vi "ConfigurePerCellMotionAnalysis.vi"(4 "Scan Settings (um)":T1={"XStart"=1, "XEnd"=1, "XNum"=1, "YStart"=1, "YEnd"=1, "YNum"=1, "ZStart"=1, "ZEnd"=1, "ZNum"=1}, 5 "Points Selected":i32, 6 "Scan Settings":T1={"XStart"=1, "XEnd"=1, "XNum"=1, "YStart"=1, "YEnd"=1, "YNum"=1, "ZStart"=1, "ZEnd"=1, "ZNum"=1}, 7 "Sampling Structure":u16(ring) items=["Cube Vertices"], 8 "error in (no error)":errorcluster, 9 "Per Cell Motion Analysis":bool, 10 "In Points":i32[][](array[numeric]), 11 "AODAcq in":refnum<class "AODAcq.lvclass">) -> (0 "error out":errorcluster, 1 "Additional Points":i32, 2 "Out Points":i32[][](array[numeric]), 3 "AODAcq out":refnum<class "AODAcq.lvclass">)   [LabVIEW 2014, in "AODAcq.lvclass"]
uses:
  AODAcq.lvclass
  Cube Vertices.vi
panel:
  # "On"
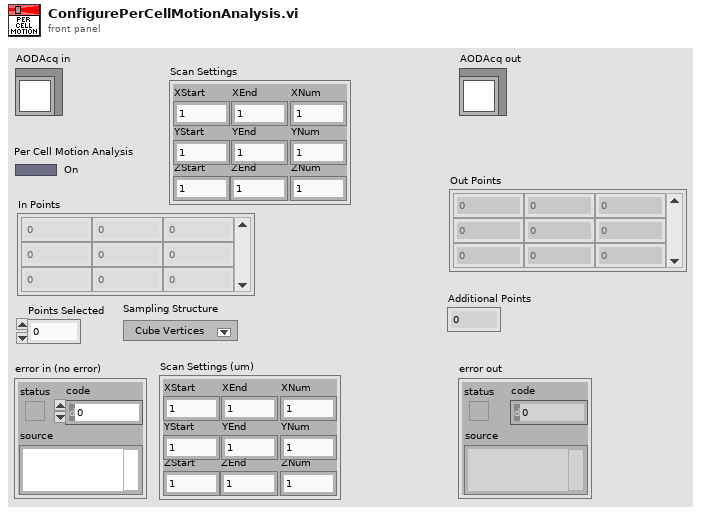
[diagram p1: front panel]
types:
  T1 = cluster{"XStart":i32, "XEnd":i32, "XNum":i32, "YStart":i32, "YEnd":i32, "YNum":i32, "ZStart":i32, "ZEnd":i32, "ZNum":i32}
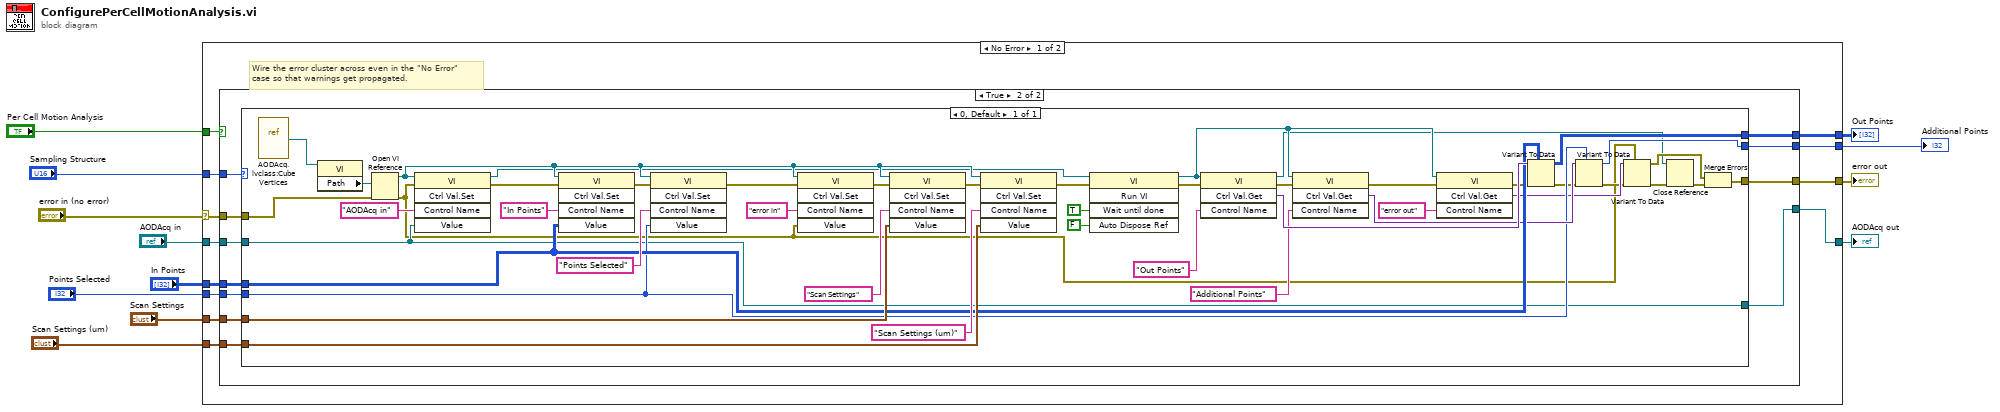
[diagram p0: block diagram]
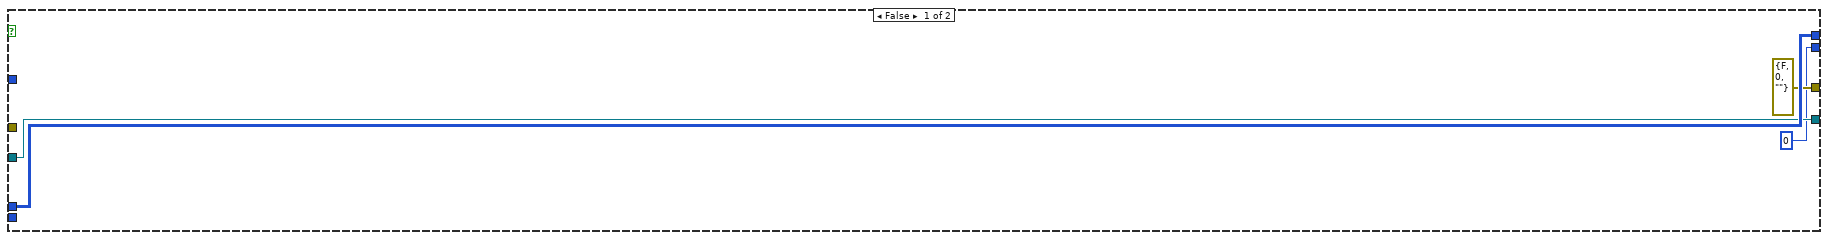
[diagram p2: hidden frame]
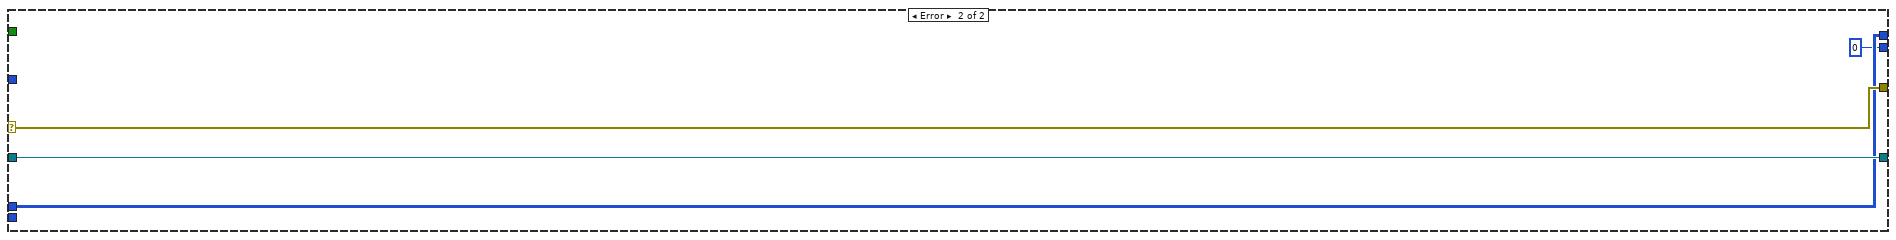
[diagram p3: hidden frame]
diagram:
  n1 = case shown="No Error" "error in (no error)" {
    selector: "error in (no error)" -> [w15 w88]
    tunnel: [w16 w88] -> w11
    tunnel: [w17 w87] -> w9
    tunnel: "AODAcq in" -> [w18 w87]
    tunnel: "Per Cell Motion Analysis" -> [w24 _]
    tunnel: "In Points" -> [w21 w86]
    tunnel: "Points Selected" -> [w23 _]
    tunnel: "Sampling Structure" -> [w22 _]
    tunnel: [w20 w86] -> w4
    tunnel: "Scan Settings" -> [w19 _]
    tunnel: "Scan Settings (um)" -> [w14 _]
    tunnel: [w13 0 ("Additional Points")] -> w1
    frame No Error {
      # "Wire the error cluster across even in the \"No Error\"\ncase so that warnings get propagated."
      n2 = case shown="True" w24 {
        tunnel: w23 -> [_ w39]
        tunnel: w22 -> [_ w38]
        tunnel: w21 -> [w28 w37]
        tunnel: [w28 w36] -> w20
        tunnel: w19 -> [_ w35]
        tunnel: w18 -> [w27 w34]
        tunnel: [w27 w29] -> w17
        tunnel: [errorcluster {"status"=FALSE, "code"=0, "source"=""} ("error out") w33] -> w16
        tunnel: w15 -> [_ w32]
        tunnel: w14 -> [_ w31]
        tunnel: [0 ("Additional Points") w30] -> w13
        frame False {
        }
        frame True {
          n3 = case shown="0, Default" w38 {
            tunnel: w39 -> [w60]
            tunnel: [w63] -> w36
            tunnel: w37 -> [w64]
            tunnel: w35 -> [w77]
            tunnel: w34 -> [w46]
            tunnel: [w47] -> w33
            tunnel: w32 -> [w43]
            tunnel: w31 -> [w75]
            tunnel: [w59] -> w30
            tunnel: [w46] -> w29
            frame 0, Default {
              n4 = vi-ref "AODAcq.lvclass:Cube Vertices.vi"() -> (w40:refnum<vi>)
              n5 = property class="VI"(reference=w40) -> ("Path"=w84:path)  [unwired: 1 in, 2 out]
              n6 = Open VI Reference(vi path=w84, error in (no error)=w43) -> (vi reference=w82:refnum<vi>, error out=w42:errorcluster)  [unwired: 4 in]
              n7 = invoke class="VI" method="Ctrl Val.Set"(reference=w82, error in=w42, "Control Name"="AODAcq in", "Value"=w46) -> (reference out=w74:refnum<vi>, error out=w71:errorcluster)  [unwired: 1 in, 3 out]
              n8 = invoke class="VI" method="Ctrl Val.Set"(reference=w82, error in=w71, "Control Name"="In Points", "Value"=w64) -> (error out=w70:errorcluster)  [unwired: 1 in, 4 out]
              n9 = invoke class="VI" method="Ctrl Val.Set"(reference=w82, error in=w70, "Control Name"="Points Selected", "Value"=w60) -> (error out=w69:errorcluster)  [unwired: 1 in, 4 out]
              n10 = invoke class="VI" method="Ctrl Val.Set"(reference=w82, error in=w69, "Control Name"="error in", "Value"=w42) -> (error out=w68:errorcluster)  [unwired: 1 in, 4 out]
              n11 = invoke class="VI" method="Ctrl Val.Set"(reference=w82, error in=w68, "Control Name"="Scan Settings", "Value"=w77) -> (error out=w67:errorcluster)  [unwired: 1 in, 4 out]
              n12 = invoke class="VI" method="Ctrl Val.Set"(reference=w82, error in=w67, "Control Name"="Scan Settings (um)", "Value"=w75) -> (error out=w56:errorcluster)  [unwired: 1 in, 4 out]
              n13 = invoke class="VI" method="Run VI"(reference=w74, error in=w56, "Wait until done"=TRUE ("Wait Until Done"), "Auto Dispose Ref"=FALSE ("Auto Dispose Reference")) -> (reference out=w53:refnum<vi>, error out=w45:errorcluster)  [unwired: 1 in, 3 out]
              n14 = invoke class="VI" method="Ctrl Val.Get"(reference=w53, error in=w45, "Control Name"="Out Points") -> (reference out=w44:refnum<vi>, error out=w55:errorcluster, "Get Control Value Variant"=w65:variant)  [unwired: 1 in, 1 out]
              n15 = invoke class="VI" method="Ctrl Val.Get"(reference=w53, error in=w55, "Control Name"="Additional Points") -> (error out=w54:errorcluster, "Get Control Value Variant"=w61:variant)  [unwired: 1 in, 2 out]
              n16 = invoke class="VI" method="Ctrl Val.Get"(reference=w53, error in=w54, "Control Name"="error out") -> (error out=w41:errorcluster, "Get Control Value Variant"=w57:variant)  [unwired: 1 in, 2 out]
              n17 = Variant To Data(error in=w41, type=w64, Variant=w65) -> (data=w63:i32[][], error out=w52:errorcluster)
              n18 = Variant To Data(error in=w52, type=w60, Variant=w61) -> (data=w59:i32, error out=w51:errorcluster)
              n19 = Variant To Data(error in=w51, type=w42, Variant=w57) -> (data=w49:errorcluster, error out=w50:errorcluster)
              n20 = Close Reference(reference=w44, error in (no error)=w50) -> (error out=w48:errorcluster)
              n21 = Merge Errors(w49, w48) -> (w47:errorcluster)
            }
          }
        }
      }
    }
    frame Error {
    }
  }
  "error out" <- w11
  "AODAcq out" <- w9
  "Out Points" <- w4
  "Additional Points" <- w1
